vi "MRB_set.vi"(7 "set_point":dbl min=0.0 max=100.0 step=0.1 format="%.1f", 8 "err_in":errorcluster, 11 "visa_in":refnum<visa-resource-name>) -> (0 "err_out":errorcluster, 2 "result":dbl, 3 "visa_out":refnum<visa-resource-name>, 4 "status":bool)   [LabVIEW 2019]
panel:
  out "read count":u32
  out "write count":u32
  out "command":string
  out "string":string
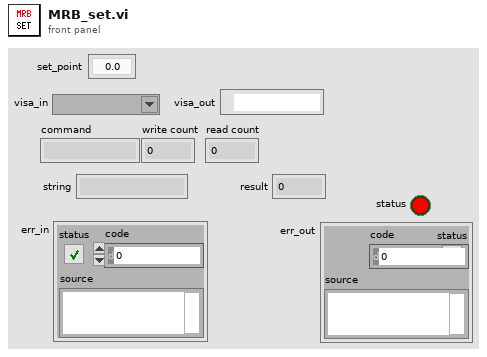
[diagram p1: front panel]
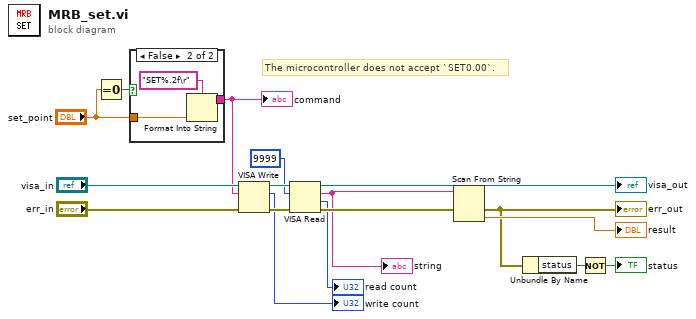
[diagram p0: block diagram]
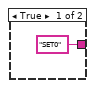
[diagram p2: hidden frame]
diagram:
  # "The microcontroller does not accept `SET0.00`."
  n1 = Equal To 0?(x="set_point") -> (x = 0?=w1:bool)
  n2 = case shown="False" w1 {
    tunnel: ["SET0" w20] -> w5
    tunnel: "set_point" -> [_ w19]
    frame True {
    }
    frame False {
      n3 = Format Into String(format string="SET%.2f\r", w19) -> (resulting string=w20:string)  [unwired: 2 in, 1 out]
    }
  }
  "command" <- w5
  n4 = VISA Write(VISA resource name="visa_in", write buffer=w5, error in (no error)="err_in") -> (VISA resource name out=w17:refnum<visa-resource-name>, return count=→"write count":u32, error out=w16:errorcluster)
  n5 = VISA Read(VISA resource name=w17, byte count=u32 9999, error in (no error)=w16) -> (VISA resource name out=→"visa_out":refnum<visa-resource-name>, read buffer=w6:string, return count=→"read count":u32, error out=w10:errorcluster)
  "string" <- w6
  n6 = Scan From String(input string=w6, error in=w10) -> (error out=w9:errorcluster, output 1=→"result":dbl)  [unwired: 3 in, 2 out]
  "err_out" <- w9
  n7 = Unbundle By Name(w9) -> ("status"=w8:bool)
  n8 = Not(x=w8) -> (.not. x?=→"status":bool)
